vi "AutoRun.vi"() -> ()   [LabVIEW 2012]
uses:
  <vilib>/Utility/error.llb/whitespace.ctl
  resultShow.vi
panel:
  in  "布尔":bool
  in  "stepECUbracket":string
  out "毫秒计时值":u32
  in  "stepMotor/ECU":string
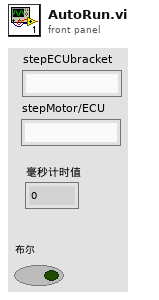
[diagram p1: front panel]
types:
  T1 = cluster{"takesTime":refnum<vi>, "userStatus":refnum<vi>, "userName":refnum<vi>, "connectionMode":refnum<vi>, "productsName":refnum<vi>, "rigStatus":refnum<vi>, "管柱码":refnum<vi>, "电机码":refnum<vi>, "控制器码":refnum<vi>, "rigStatus 2":refnum<vi>}
  T2 = typedef "whitespace.ctl" = u16
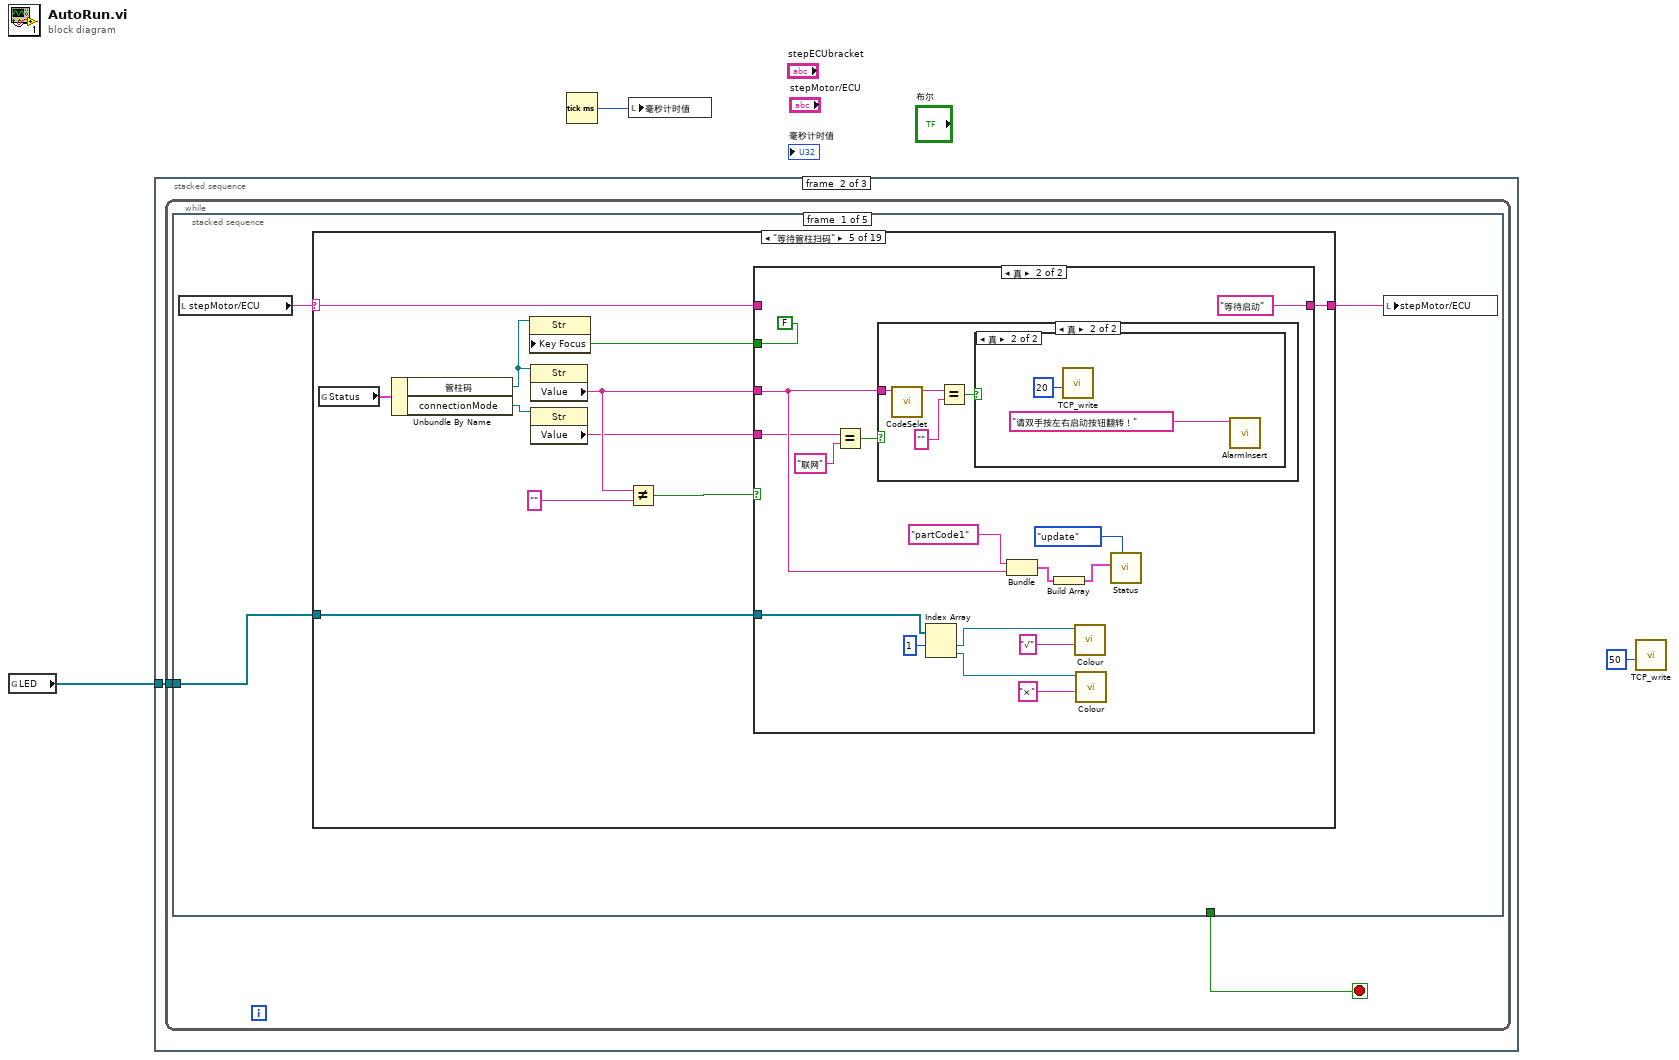
[diagram p0: block diagram]
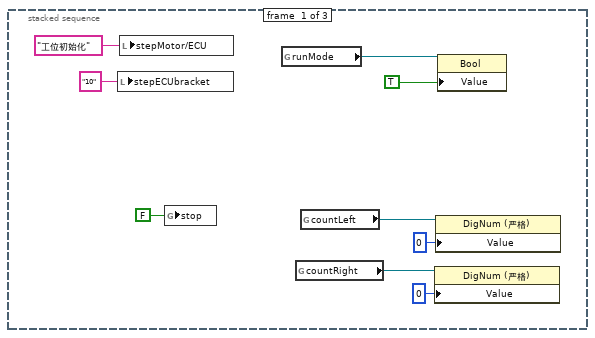
[diagram p2: hidden frame]
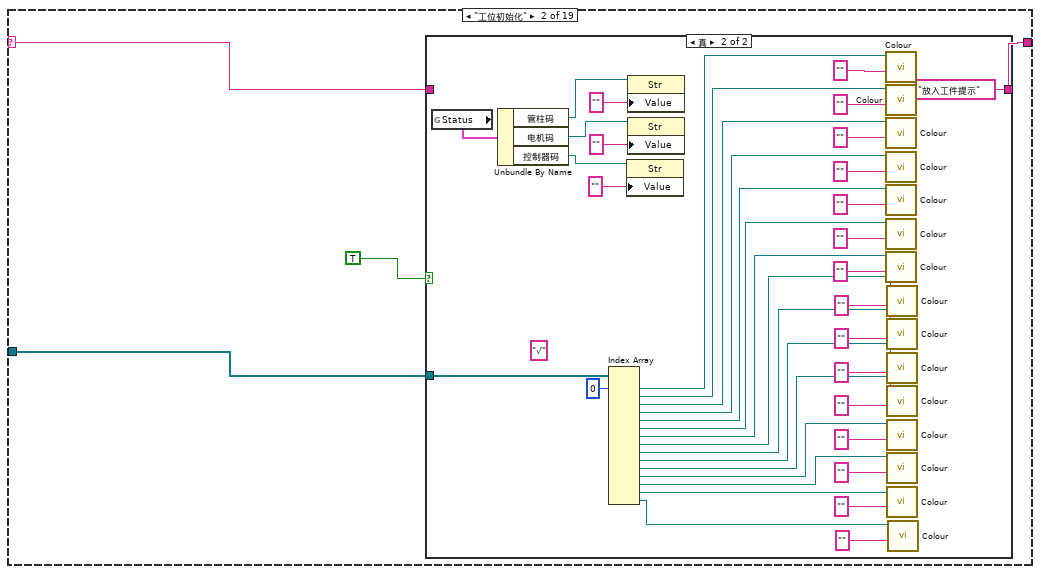
[diagram p4: hidden frame]
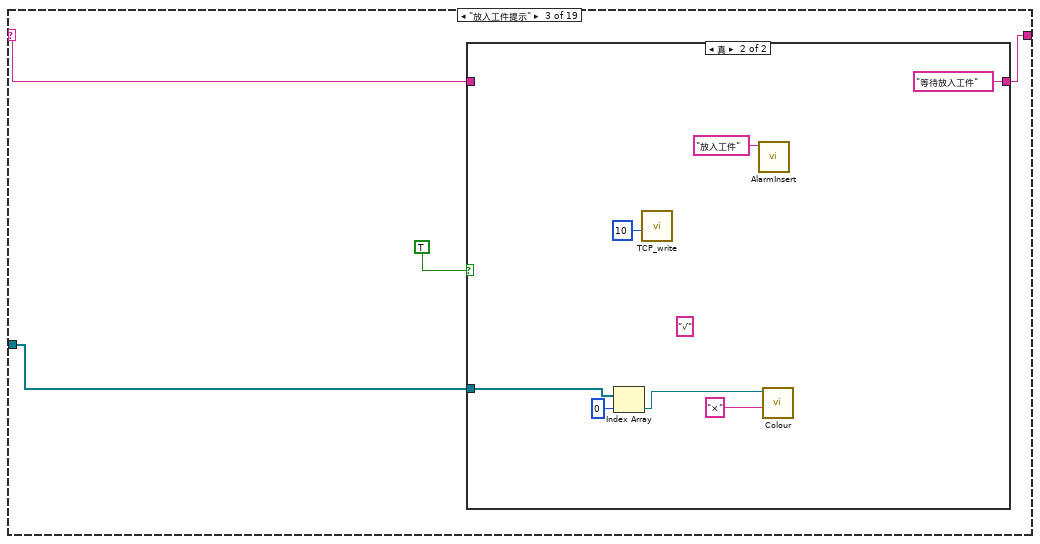
[diagram p6: hidden frame]
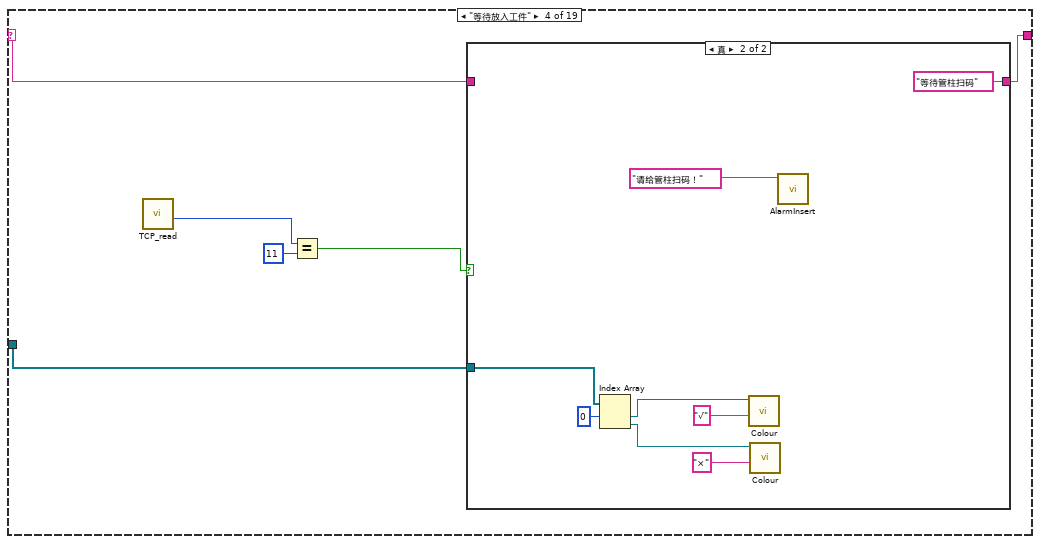
[diagram p8: hidden frame]
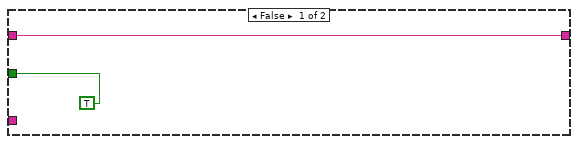
[diagram p10: hidden frame]
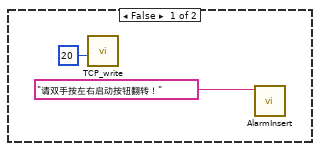
[diagram p11: hidden frame]
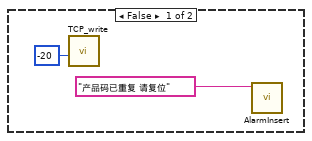
[diagram p12: hidden frame]
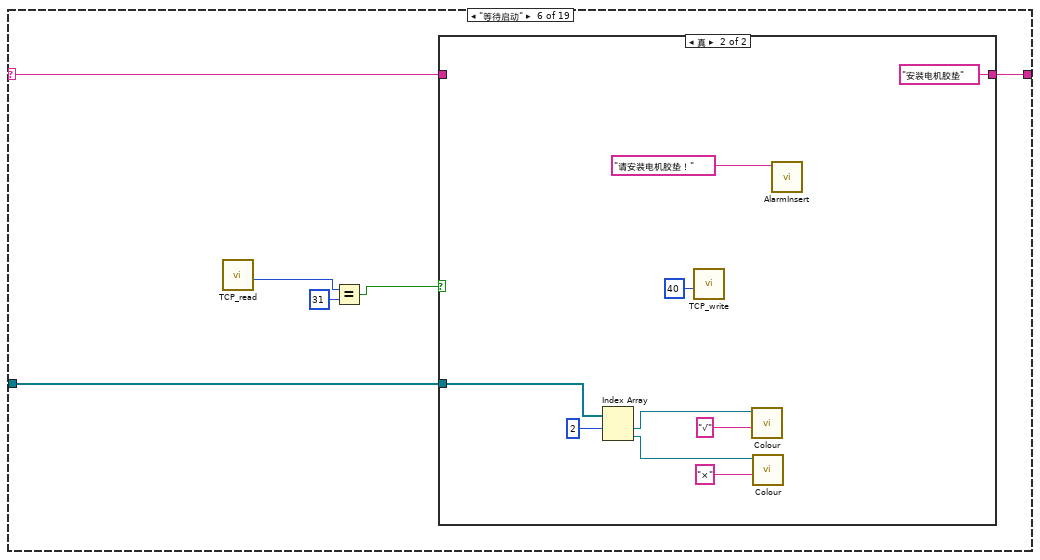
[diagram p13: hidden frame]
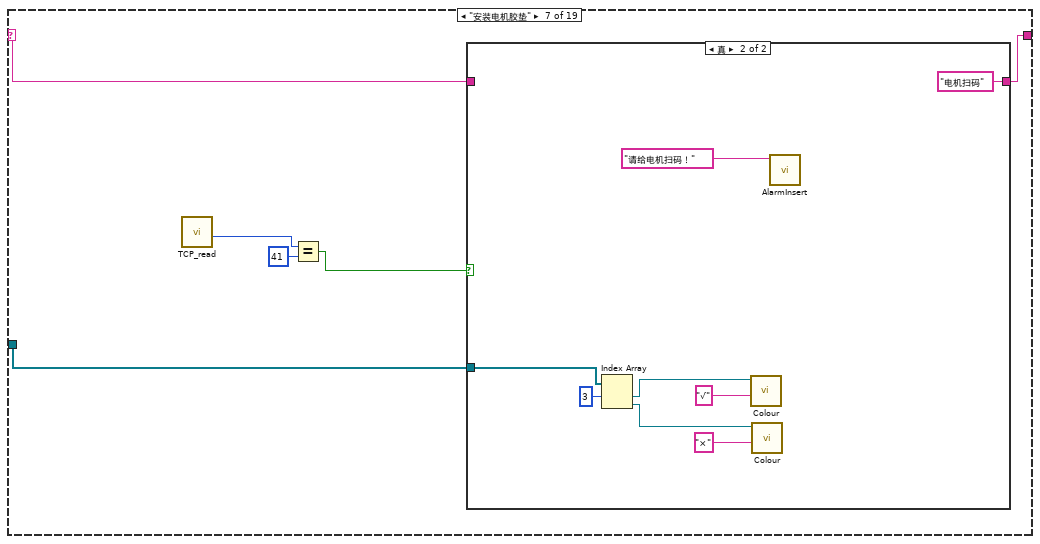
[diagram p15: hidden frame]
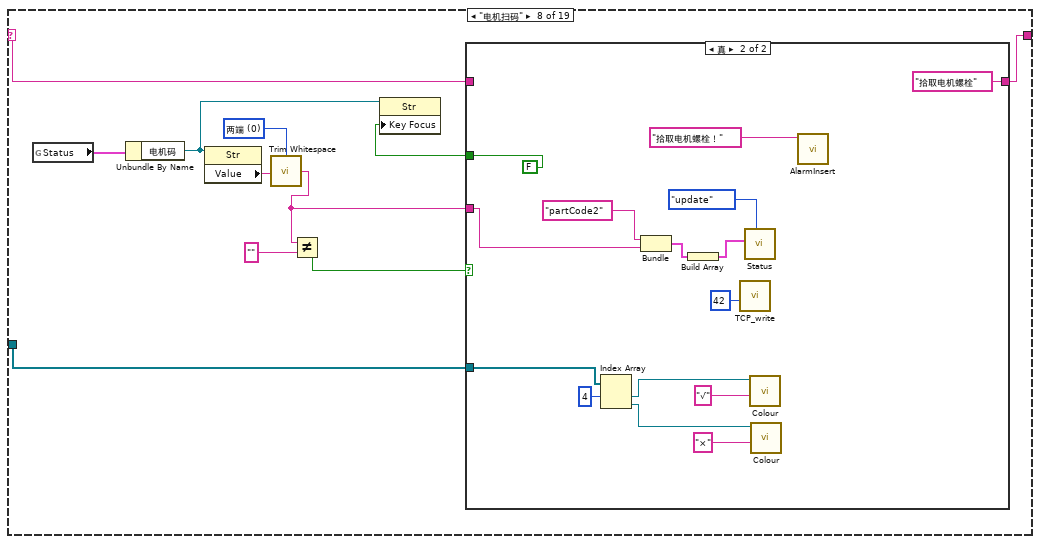
[diagram p17: hidden frame]
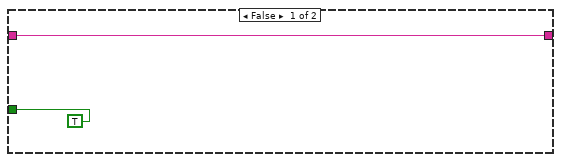
[diagram p18: hidden frame]
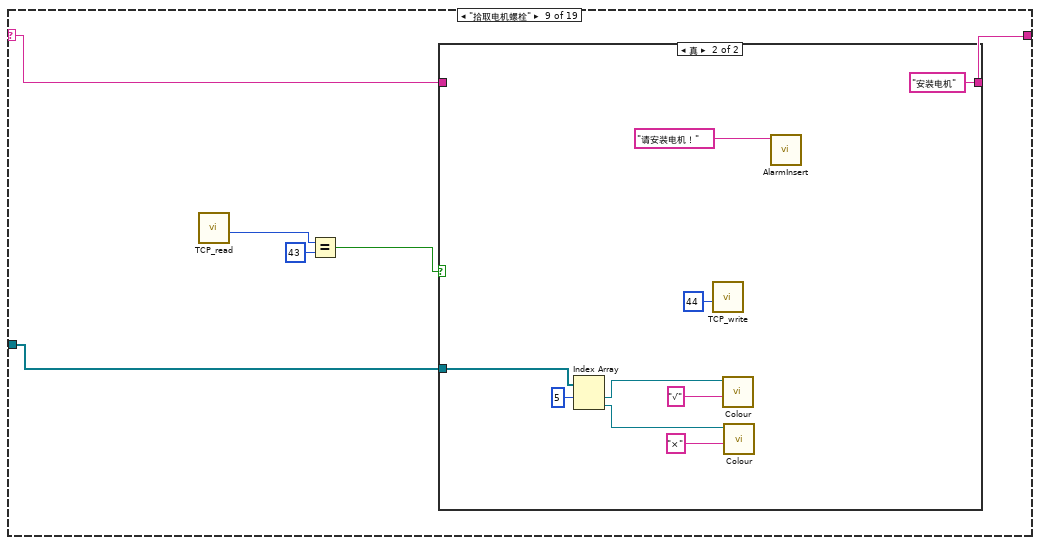
[diagram p19: hidden frame]
diagram:
  n1 = global read "resultShow.vi" "LED"() -> (w3:refnum<vi>[])
  n2 = stacked-sequence {
    tunnel: w3 -> [_ w13 _]
    frame #0 {
      n3 = local write "stepECUbracket"("10" ("step")) -> ()
      n4 = local write "stepMotor/ECU"("工位初始化" ("step")) -> ()
      n5 = global write "全局 3.vi" "stop"(FALSE ("布尔 2")) -> ()
      n6 = global read "resultShow.vi" "runMode"() -> (w9:refnum<vi>)
      n7 = global read "resultShow.vi" "countRight"() -> (w7:refnum<vi>)
      n8 = global read "resultShow.vi" "countLeft"() -> (w4:refnum<vi>)
      n9 = property class="DigNum (严格)"(reference=w7, "Value"=u32 0 ("值")) -> ()  [unwired: 1 in, 2 out]
      n10 = property class="DigNum (严格)"(reference=w4, "Value"=u32 0 ("值")) -> ()  [unwired: 1 in, 2 out]
      n11 = property class="Bool"(reference=w9, "Value"=TRUE ("m")) -> ()  [unwired: 1 in, 2 out]
    }
    frame #1 {
      n12 = while {
        tunnel: w13 -> [w14]
        stop <- w15 stop-if-true
        n13 = stacked-sequence {
          tunnel: [_ _ _ _ w510] -> w15
          tunnel: w14 -> [w17 _ _ w410 _]
          frame #0 {
            n14 = local read "stepMotor/ECU"() -> (w16:string)
            n15 = case shown="\"等待管柱扫码\"" w16 {
              selector: w16 -> [w19 w22 w67 w81 w101 w135 w151 w171 w193 w210 w224 w240 w256 w277 w299 w316 w329 w347 w370]
              tunnel: [w19 w23 w68 w82 w102 w136 w152 w169 w195 w211 w222 w238 w254 w272 w300 w315 w327 w348 w371] -> w18
              tunnel: w17 -> [_ w21 w66 w77 w100 w131 w147 w170 w194 w206 w223 w239 w255 w276 w298 w314 w328 w343 w366]
              frame "假", Default {
              }
              frame "工位初始化" {
                n16 = case shown="真" TRUE {
                  tunnel: [w24 "放入工件提示"] -> w23
                  tunnel: w22 -> [w24 _]
                  tunnel: w21 -> [_ w62]
                  frame False {
                  }
                  frame True {
                    (unwired) "√" ("元素")
                    n17 = global read "resultShow.vi" "Status"() -> (w35:T1)
                    n18 = Unbundle By Name(w35) -> ("管柱码"=w34:refnum<vi>, "电机码"=w31:refnum<vi>, "控制器码"=w29:refnum<vi>)
                    n19 = Index Array(array=w62, index #1=0 ("索引")) -> (element #1=w54:refnum<vi>, element #2=w53:refnum<vi>, element #3=w52:refnum<vi>, element #4=w51:refnum<vi>, element #5=w50:refnum<vi>, element #6=w49:refnum<vi>, element #7=w48:refnum<vi>, element #8=w41:refnum<vi>, element #9=w40:refnum<vi>, element #10=w39:refnum<vi>, element #11=w38:refnum<vi>, element #12=w37:refnum<vi>, element #13=w36:refnum<vi>, element #14=w27:refnum<vi>, element #15=w25:refnum<vi>)  [unwired: 14 in]
                    n20 = property class="Str"(reference=w29, "Value"="") -> ()  [unwired: 1 in, 2 out]
                    n21 = property class="Str"(reference=w34, "Value"="") -> ()  [unwired: 1 in, 2 out]
                    n22 = property class="Str"(reference=w31, "Value"="") -> ()  [unwired: 1 in, 2 out]
                    n23 = call "Colour.vi"("result"="" ("元素"), "colourRef"=w54) -> ()  [unwired: 9 in, 1 out]
                    n24 = call "Colour.vi"("result"="" ("元素"), "colourRef"=w53) -> ()  [unwired: 9 in, 1 out]
                    n25 = call "Colour.vi"("result"="" ("元素"), "colourRef"=w52) -> ()  [unwired: 9 in, 1 out]
                    n26 = call "Colour.vi"("result"="" ("元素"), "colourRef"=w51) -> ()  [unwired: 9 in, 1 out]
                    n27 = call "Colour.vi"("result"="" ("元素"), "colourRef"=w50) -> ()  [unwired: 9 in, 1 out]
                    n28 = call "Colour.vi"("result"="" ("元素"), "colourRef"=w49) -> ()  [unwired: 9 in, 1 out]
                    n29 = call "Colour.vi"("result"="" ("元素"), "colourRef"=w48) -> ()  [unwired: 9 in, 1 out]
                    n30 = call "Colour.vi"("result"="" ("元素"), "colourRef"=w41) -> ()  [unwired: 9 in, 1 out]
                    n31 = call "Colour.vi"("result"="" ("元素"), "colourRef"=w40) -> ()  [unwired: 9 in, 1 out]
                    n32 = call "Colour.vi"("result"="" ("元素"), "colourRef"=w39) -> ()  [unwired: 9 in, 1 out]
                    n33 = call "Colour.vi"("result"="" ("元素"), "colourRef"=w38) -> ()  [unwired: 9 in, 1 out]
                    n34 = call "Colour.vi"("result"="" ("元素"), "colourRef"=w37) -> ()  [unwired: 9 in, 1 out]
                    n35 = call "Colour.vi"("result"="" ("元素"), "colourRef"=w36) -> ()  [unwired: 9 in, 1 out]
                    n36 = call "Colour.vi"("result"="" ("元素"), "colourRef"=w27) -> ()  [unwired: 9 in, 1 out]
                    n37 = call "Colour.vi"("result"="" ("元素"), "colourRef"=w25) -> ()  [unwired: 9 in, 1 out]
                  }
                }
              }
              frame "放入工件提示" {
                n38 = case shown="真" TRUE {
                  tunnel: [w69 "等待放入工件"] -> w68
                  tunnel: w67 -> [w69 _]
                  tunnel: w66 -> [_ w72]
                  frame False {
                  }
                  frame True {
                    (unwired) "√" ("元素")
                    n39 = Index Array(array=w72, index=0 ("索引")) -> (element=w74:refnum<vi>)
                    n40 = call "TCP_write.vi"("写入数据"=i8 10) -> ()  [unwired: 11 in]
                    n41 = call "AlarmInsert.vi"("消息名"="放入工件") -> ()  [unwired: 11 in]
                    n42 = call "Colour.vi"("result"="×" ("元素"), "colourRef"=w74) -> ()  [unwired: 9 in, 1 out]
                  }
                }
              }
              frame "等待放入工件" {
                n43 = call "TCP_read.vi"() -> ("元素"=w80:i8)  [unwired: 10 in, 1 out]
                n44 = Equal?(x=w80, y=i8 11) -> (x = y?=w78:bool)
                n45 = case shown="真" w78 {
                  tunnel: [w83 "等待管柱扫码"] -> w82
                  tunnel: w81 -> [w83 _]
                  tunnel: w77 -> [_ w84]
                  frame False {
                  }
                  frame True {
                    n46 = Index Array(array=w84, index #1=0 ("索引")) -> (element #1=w88:refnum<vi>, element #2=w85:refnum<vi>)  [unwired: 1 in]
                    n47 = call "Colour.vi"("result"="√" ("元素"), "colourRef"=w88) -> ()  [unwired: 9 in, 1 out]
                    n48 = call "Colour.vi"("result"="×" ("元素"), "colourRef"=w85) -> ()  [unwired: 9 in, 1 out]
                    n49 = call "AlarmInsert.vi"("消息名"="请给管柱扫码！" ("string_5")) -> ()  [unwired: 11 in]
                  }
                }
              }
              frame "等待管柱扫码" {
                n50 = global read "resultShow.vi" "Status"() -> (w99:T1)
                n51 = Unbundle By Name(w99) -> ("管柱码"=w96:refnum<vi>, "connectionMode"=w93:refnum<vi>)
                n52 = property class="Str"(reference=w96) -> ("Value"=w94:string)  [unwired: 1 in, 2 out]
                n53 = property class="Str"(reference=w93) -> ("Value"=w92:string)  [unwired: 1 in, 2 out]
                n54 = Not Equal?(x=w94, y="") -> (x != y?=w98:bool)
                n55 = case shown="真" w98 {
                  tunnel: [w104 "等待启动"] -> w102
                  tunnel: w101 -> [w104 _]
                  tunnel: w100 -> [_ w114]
                  tunnel: [TRUE FALSE] -> w95
                  tunnel: w94 -> [_ w108]
                  tunnel: w92 -> [_ w105]
                  frame False {
                  }
                  frame True {
                    n56 = Equal?(x=w105, y="联网") -> (x = y?=w107:bool)
                    n57 = case shown="真" w107 {
                      tunnel: w108 -> [_ w126]
                      frame False {
                        n58 = call "TCP_write.vi"("写入数据"=i8 20) -> ()  [unwired: 11 in]
                        n59 = call "AlarmInsert.vi"("消息名"="请双手按左右启动按钮翻转！" ("string_5")) -> ()  [unwired: 11 in]
                      }
                      frame True {
                        n60 = call "CodeSelet.vi"("parameter name"=w126) -> ("readData"=w125:string)  [unwired: 10 in]
                        n61 = Equal?(x=w125, y="") -> (x = y?=w124:bool)
                        n62 = case shown="真" w124 {
                          frame False {
                            n63 = call "TCP_write.vi"("写入数据"=i8 -20) -> ()  [unwired: 11 in]
                            n64 = call "AlarmInsert.vi"("消息名"="产品码已重复 请复位" ("string_5")) -> ()  [unwired: 11 in]
                          }
                          frame True {
                            n65 = call "TCP_write.vi"("写入数据"=i8 20) -> ()  [unwired: 11 in]
                            n66 = call "AlarmInsert.vi"("消息名"="请双手按左右启动按钮翻转！" ("string_5")) -> ()  [unwired: 11 in]
                          }
                        }
                      }
                    }
                    n67 = Index Array(array=w114, index #1=1 ("索引")) -> (element #1=w118:refnum<vi>, element #2=w115:refnum<vi>)  [unwired: 1 in]
                    n68 = Bundle("元素"="partCode1", "Value"=w108) -> (w110:cluster{"元素":string, "Value":string})  [unwired: 1 in]
                    n69 = Build Array(w110) -> (w111:cluster{"元素":string, "Value":string}[])
                    n70 = call "Colour.vi"("result"="√" ("元素"), "colourRef"=w118) -> ()  [unwired: 9 in, 1 out]
                    n71 = call "Colour.vi"("result"="×" ("元素"), "colourRef"=w115) -> ()  [unwired: 9 in, 1 out]
                    n72 = call "Status.vi"("模式"=enum16{"select", "insert", "update", "delete"}."update", "nameData"=w111) -> ()  [unwired: 9 in, 1 out]
                  }
                }
                n73 = property class="Str"(reference=w96, "Key Focus"=w95) -> ()  [unwired: 1 in, 2 out]
              }
              frame "等待启动" {
                n74 = call "TCP_read.vi"() -> ("元素"=w134:i8)  [unwired: 10 in, 1 out]
                n75 = Equal?(x=w134, y=i8 31) -> (x = y?=w132:bool)
                n76 = case shown="真" w132 {
                  tunnel: [w137 "安装电机胶垫"] -> w136
                  tunnel: w135 -> [w137 _]
                  tunnel: w131 -> [_ w139]
                  frame False {
                  }
                  frame True {
                    n77 = Index Array(array=w139, index #1=2 ("索引")) -> (element #1=w143:refnum<vi>, element #2=w140:refnum<vi>)  [unwired: 1 in]
                    n78 = call "TCP_write.vi"("写入数据"=i8 40) -> ()  [unwired: 11 in]
                    n79 = call "Colour.vi"("result"="√" ("元素"), "colourRef"=w143) -> ()  [unwired: 9 in, 1 out]
                    n80 = call "Colour.vi"("result"="×" ("元素"), "colourRef"=w140) -> ()  [unwired: 9 in, 1 out]
                    n81 = call "AlarmInsert.vi"("消息名"="请安装电机胶垫！" ("string_5")) -> ()  [unwired: 11 in]
                  }
                }
              }
              frame "安装电机胶垫" {
                n82 = call "TCP_read.vi"() -> ("元素"=w150:i8)  [unwired: 10 in, 1 out]
                n83 = Equal?(x=w150, y=i8 41) -> (x = y?=w148:bool)
                n84 = case shown="真" w148 {
                  tunnel: [w153 "电机扫码"] -> w152
                  tunnel: w151 -> [w153 _]
                  tunnel: w147 -> [_ w154]
                  frame False {
                  }
                  frame True {
                    n85 = Index Array(array=w154, index #1=3 ("索引")) -> (element #1=w158:refnum<vi>, element #2=w155:refnum<vi>)  [unwired: 1 in]
                    n86 = call "Colour.vi"("result"="√" ("元素"), "colourRef"=w158) -> ()  [unwired: 9 in, 1 out]
                    n87 = call "Colour.vi"("result"="×" ("元素"), "colourRef"=w155) -> ()  [unwired: 9 in, 1 out]
                    n88 = call "AlarmInsert.vi"("消息名"="请给电机扫码！" ("string_5")) -> ()  [unwired: 11 in]
                  }
                }
              }
              frame "电机扫码" {
                w162 = T2 0 items=["两端", "字符串首端", "字符串末端"] ("location (both)")
                n89 = global read "resultShow.vi" "Status"() -> (w167:T1)
                n90 = Unbundle By Name(w167) -> ("电机码"=w166:refnum<vi>)
                n91 = property class="Str"(reference=w166) -> ("Value"=w164:string)  [unwired: 1 in, 2 out]
                n92 = call <vilib>:"Trim Whitespace.vi"("string"=w164, "location (both)"=w162) -> ("trimmed string"=w163:string)
                n93 = Not Equal?(x=w163, y="") -> (x != y?=w172:bool)
                n94 = case shown="真" w172 {
                  tunnel: [w174 "拾取电机螺栓"] -> w169
                  tunnel: w171 -> [w174 _]
                  tunnel: w170 -> [_ w181]
                  tunnel: [TRUE FALSE] -> w165
                  tunnel: w163 -> [_ w175]
                  frame False {
                  }
                  frame True {
                    n95 = Index Array(array=w181, index #1=4 ("索引")) -> (element #1=w185:refnum<vi>, element #2=w182:refnum<vi>)  [unwired: 1 in]
                    n96 = Bundle("元素"="partCode2", "trimmed string"=w175) -> (w177:cluster{"元素":string, "trimmed string":string})  [unwired: 1 in]
                    n97 = Build Array(w177) -> (w178:cluster{"元素":string, "trimmed string":string}[])
                    n98 = call "TCP_write.vi"("写入数据"=i8 42) -> ()  [unwired: 11 in]
                    n99 = call "Status.vi"("模式"=enum16{"select", "insert", "update", "delete"}."update", "nameData"=w178) -> ()  [unwired: 9 in, 1 out]
                    n100 = call "Colour.vi"("result"="√" ("元素"), "colourRef"=w185) -> ()  [unwired: 9 in, 1 out]
                    n101 = call "Colour.vi"("result"="×" ("元素"), "colourRef"=w182) -> ()  [unwired: 9 in, 1 out]
                    n102 = call "AlarmInsert.vi"("消息名"="拾取电机螺栓！" ("string_5")) -> ()  [unwired: 11 in]
                  }
                }
                n103 = property class="Str"(reference=w166, "Key Focus"=w165) -> ()  [unwired: 1 in, 2 out]
              }
              frame "拾取电机螺栓" {
                n104 = call "TCP_read.vi"() -> ("元素"=w192:i8)  [unwired: 10 in, 1 out]
                n105 = Equal?(x=w192, y=i8 43) -> (x = y?=w190:bool)
                n106 = case shown="真" w190 {
                  tunnel: [w196 "安装电机"] -> w195
                  tunnel: w193 -> [w196 _]
                  tunnel: w194 -> [_ w197]
                  frame False {
                  }
                  frame True {
                    n107 = Index Array(array=w197, index #1=5 ("索引")) -> (element #1=w201:refnum<vi>, element #2=w198:refnum<vi>)  [unwired: 1 in]
                    n108 = call "TCP_write.vi"("写入数据"=i8 44) -> ()  [unwired: 11 in]
                    n109 = call "Colour.vi"("result"="√" ("元素"), "colourRef"=w201) -> ()  [unwired: 9 in, 1 out]
                    n110 = call "Colour.vi"("result"="×" ("元素"), "colourRef"=w198) -> ()  [unwired: 9 in, 1 out]
                    n111 = call "AlarmInsert.vi"("消息名"="请安装电机！" ("string_5")) -> ()  [unwired: 11 in]
                  }
                }
              }
              frame "安装电机" {
                n112 = call "TCP_read.vi"() -> ("元素"=w209:i8)  [unwired: 10 in, 1 out]
                n113 = Equal?(x=w209, y=i8 45) -> (x = y?=w207:bool)
                n114 = case shown="真" w207 {
                  tunnel: [w212 "涂电机色标"] -> w211
                  tunnel: w210 -> [w212 _]
                  tunnel: w206 -> [_ w213]
                  frame False {
                  }
                  frame True {
                    n115 = Index Array(array=w213, index #1=6 ("索引")) -> (element #1=w217:refnum<vi>, element #2=w214:refnum<vi>)  [unwired: 1 in]
                    n116 = call "TCP_write.vi"("写入数据"=i8 46) -> ()  [unwired: 11 in]
                    n117 = call "Colour.vi"("result"="√" ("元素"), "colourRef"=w217) -> ()  [unwired: 9 in, 1 out]
                    n118 = call "Colour.vi"("result"="×" ("元素"), "colourRef"=w214) -> ()  [unwired: 9 in, 1 out]
                    n119 = call "AlarmInsert.vi"("消息名"="请涂电机色标！" ("string_5")) -> ()  [unwired: 11 in]
                  }
                }
              }
              frame "涂电机色标" {
                n120 = call "TCP_read.vi"() -> ("元素"=w227:i8)  [unwired: 10 in, 1 out]
                n121 = Equal?(x=w227, y=i8 47) -> (x = y?=w225:bool)
                n122 = case shown="真" w225 {
                  tunnel: [w228 "启动平翻"] -> w222
                  tunnel: w224 -> [w228 _]
                  tunnel: w223 -> [_ w229]
                  frame False {
                  }
                  frame True {
                    n123 = Index Array(array=w229, index #1=7 ("索引")) -> (element #1=w233:refnum<vi>, element #2=w230:refnum<vi>)  [unwired: 1 in]
                    n124 = call "TCP_write.vi"("写入数据"=i8 50) -> ()  [unwired: 11 in]
                    n125 = call "Colour.vi"("result"="√" ("元素"), "colourRef"=w233) -> ()  [unwired: 9 in, 1 out]
                    n126 = call "Colour.vi"("result"="×" ("元素"), "colourRef"=w230) -> ()  [unwired: 9 in, 1 out]
                    n127 = call "AlarmInsert.vi"("消息名"="请双手按启动按钮翻转至平位" ("string_5")) -> ()  [unwired: 11 in]
                  }
                }
              }
              frame "启动平翻" {
                n128 = call "TCP_read.vi"() -> ("元素"=w241:i8)  [unwired: 10 in, 1 out]
                n129 = Equal?(x=w241, y=i8 53) -> (x = y?=w243:bool)
                n130 = case shown="真" w243 {
                  tunnel: [w244 "防错确认"] -> w238
                  tunnel: w240 -> [w244 _]
                  tunnel: w239 -> [_ w246]
                  frame False {
                  }
                  frame True {
                    n131 = Index Array(array=w246, index #1=8 ("索引")) -> (element #1=w250:refnum<vi>, element #2=w247:refnum<vi>)  [unwired: 1 in]
                    n132 = call "Colour.vi"("result"="√" ("元素"), "colourRef"=w250) -> ()  [unwired: 9 in, 1 out]
                    n133 = call "Colour.vi"("result"="×" ("元素"), "colourRef"=w247) -> ()  [unwired: 9 in, 1 out]
                    n134 = call "TCP_write.vi"("写入数据"=i8 90) -> ()  [unwired: 11 in]
                    n135 = call "AlarmInsert.vi"("消息名"="防错确认" ("string_5")) -> ()  [unwired: 11 in]
                  }
                }
              }
              frame "防错确认" {
                n136 = call "TCP_read.vi"() -> ("元素"=w257:i8)  [unwired: 10 in, 1 out]
                n137 = Equal?(x=w257, y=i8 91) -> (x = y?=w259:bool)
                n138 = case shown="真" w259 {
                  tunnel: [w260 "控制器扫码"] -> w254
                  tunnel: w256 -> [w260 _]
                  tunnel: w255 -> [_ w261]
                  frame False {
                  }
                  frame True {
                    n139 = Index Array(array=w261, index #1=9 ("索引")) -> (element #1=w265:refnum<vi>, element #2=w262:refnum<vi>)  [unwired: 1 in]
                    n140 = call "Colour.vi"("result"="√" ("元素"), "colourRef"=w265) -> ()  [unwired: 9 in, 1 out]
                    n141 = call "Colour.vi"("result"="×" ("元素"), "colourRef"=w262) -> ()  [unwired: 9 in, 1 out]
                    n142 = call "AlarmInsert.vi"("消息名"="取控制器扫码" ("string_5")) -> ()  [unwired: 11 in]
                  }
                }
              }
              frame "控制器扫码" {
                n143 = global read "resultShow.vi" "Status"() -> (w274:T1)
                n144 = Unbundle By Name(w274) -> ("控制器码"=w271:refnum<vi>)
                n145 = property class="Str"(reference=w271) -> ("Value"=w269:string)  [unwired: 1 in, 2 out]
                n146 = Not Equal?(x=w269, y="") -> (x != y?=w273:bool)
                n147 = case shown="真" w273 {
                  tunnel: [w279 "拾取控制器螺栓"] -> w272
                  tunnel: w277 -> [w279 _]
                  tunnel: w276 -> [_ w287]
                  tunnel: [TRUE FALSE] -> w270
                  tunnel: w269 -> [_ w280]
                  frame False {
                  }
                  frame True {
                    n148 = Index Array(array=w287, index #1=10 ("索引")) -> (element #1=w291:refnum<vi>, element #2=w288:refnum<vi>)  [unwired: 1 in]
                    n149 = Bundle("元素"="partCode3", "Value"=w280) -> (w282:cluster{"元素":string, "Value":string})  [unwired: 1 in]
                    n150 = Build Array(w282) -> (w283:cluster{"元素":string, "Value":string}[])
                    n151 = call "Colour.vi"("result"="√" ("元素"), "colourRef"=w291) -> ()  [unwired: 9 in, 1 out]
                    n152 = call "Colour.vi"("result"="×" ("元素"), "colourRef"=w288) -> ()  [unwired: 9 in, 1 out]
                    n153 = call "TCP_write.vi"("写入数据"=i8 54) -> ()  [unwired: 11 in]
                    n154 = call "Status.vi"("模式"=enum16{"select", "insert", "update", "delete"}."update", "nameData"=w283) -> ()  [unwired: 9 in, 1 out]
                    n155 = call "AlarmInsert.vi"("消息名"="拾取控制器螺栓" ("string_5")) -> ()  [unwired: 11 in]
                  }
                }
                n156 = property class="Str"(reference=w271, "Key Focus"=w270) -> ()  [unwired: 1 in, 2 out]
              }
              frame "拾取控制器螺栓" {
                n157 = call "TCP_read.vi"() -> ("元素"=w296:i8)  [unwired: 10 in, 1 out]
                n158 = Equal?(x=w296, y=i8 55) -> (x = y?=w295:bool)
                n159 = case shown="真" w295 {
                  tunnel: [w301 "安装控制器"] -> w300
                  tunnel: w299 -> [w301 _]
                  tunnel: w298 -> [_ w303]
                  frame False {
                  }
                  frame True {
                    n160 = Index Array(array=w303, index #1=11 ("索引")) -> (element #1=w307:refnum<vi>, element #2=w304:refnum<vi>)  [unwired: 1 in]
                    n161 = call "TCP_write.vi"("写入数据"=i8 56) -> ()  [unwired: 11 in]
                    n162 = call "Colour.vi"("result"="√" ("元素"), "colourRef"=w307) -> ()  [unwired: 9 in, 1 out]
                    n163 = call "Colour.vi"("result"="×" ("元素"), "colourRef"=w304) -> ()  [unwired: 9 in, 1 out]
                    n164 = call "AlarmInsert.vi"("消息名"="请安装控制器" ("string_5")) -> ()  [unwired: 11 in]
                  }
                }
              }
              frame "安装控制器" {
                n165 = call "TCP_read.vi"() -> ("元素"=w312:i8)  [unwired: 10 in, 1 out]
                n166 = Equal?(x=w312, y=i8 57) -> (x = y?=w311:bool)
                n167 = case shown="真" w311 {
                  tunnel: [w317 "涂控制器色标"] -> w315
                  tunnel: w316 -> [w317 _]
                  tunnel: w314 -> [_ w319]
                  frame False {
                  }
                  frame True {
                    n168 = Index Array(array=w319, index #1=12 ("索引")) -> (element #1=w323:refnum<vi>, element #2=w320:refnum<vi>)  [unwired: 1 in]
                    n169 = call "TCP_write.vi"("写入数据"=i8 60) -> ()  [unwired: 11 in]
                    n170 = call "Colour.vi"("result"="√" ("元素"), "colourRef"=w323) -> ()  [unwired: 9 in, 1 out]
                    n171 = call "Colour.vi"("result"="×" ("元素"), "colourRef"=w320) -> ()  [unwired: 9 in, 1 out]
                    n172 = call "AlarmInsert.vi"("消息名"="请涂控制器螺钉色标" ("string_5")) -> ()  [unwired: 11 in]
                  }
                }
              }
              frame "涂控制器色标" {
                n173 = call "TCP_read.vi"() -> ("元素"=w331:i8)  [unwired: 10 in, 1 out]
                n174 = Equal?(x=w331, y=i8 61) -> (x = y?=w330:bool)
                n175 = case shown="真" w330 {
                  tunnel: [w333 "80"] -> w327
                  tunnel: w329 -> [w333 _]
                  tunnel: w328 -> [_ w335]
                  frame False {
                  }
                  frame True {
                    n176 = Index Array(array=w335, index #1=13 ("索引")) -> (element #1=w339:refnum<vi>, element #2=w336:refnum<vi>)  [unwired: 1 in]
                    n177 = call "TCP_write.vi"("写入数据"=i8 70) -> ()  [unwired: 11 in]
                    n178 = call "Colour.vi"("result"="√" ("元素"), "colourRef"=w339) -> ()  [unwired: 9 in, 1 out]
                    n179 = call "Colour.vi"("result"="×" ("元素"), "colourRef"=w336) -> ()  [unwired: 9 in, 1 out]
                    n180 = call "AlarmInsert.vi"("消息名"="请取出工件" ("string_5")) -> ()  [unwired: 11 in]
                  }
                }
              }
              frame "80" {
                n181 = call "TCP_read.vi"() -> ("元素"=w346:i8)  [unwired: 10 in, 1 out]
                n182 = Equal?(x=w346, y=i8 71) -> (x = y?=w344:bool)
                n183 = case shown="真" w344 {
                  tunnel: [w349 "90"] -> w348
                  tunnel: w347 -> [w349 _]
                  tunnel: w343 -> [_ w350]
                  frame False {
                  }
                  frame True {
                    n184 = local read "毫秒计时值"() -> (w357:u32)
                    n185 = Tick Count (ms)() -> (millisecond timer value=w362:u32)
                    n186 = Index Array(array=w350, index #1=13 ("索引")) -> (element #1=w354:refnum<vi>, element #2=w351:refnum<vi>)  [unwired: 1 in]
                    n187 = Subtract(x=w362, y=w357) -> (x-y=w361:u32)
                    n188 = Divide(x=w361, y=u32 1000) -> (x/y=w359:dbl)
                    n189 = To Time Stamp(1:w359) -> (0:w358:timestamp)
                    n190 = call "Colour.vi"("result"="√" ("元素"), "colourRef"=w354) -> ()  [unwired: 9 in, 1 out]
                    n191 = call "Colour.vi"("result"="×" ("元素"), "colourRef"=w351) -> ()  [unwired: 9 in, 1 out]
                    n192 = Format Date/Time String(seconds (now)=w358) -> (date/time string=w356:string)  [unwired: 2 in]
                    n193 = call "TCP_write.vi"("写入数据"=i8 80) -> ()  [unwired: 11 in]
                    n194 = call "AlarmInsert.vi"("takesTime"=w356, "消息名"="完成取回工件！" ("string_5")) -> ()  [unwired: 10 in]
                  }
                }
              }
              frame "90" {
                n195 = call "TCP_read.vi"() -> ("元素"=w369:i8)  [unwired: 10 in, 1 out]
                n196 = Equal?(x=w369, y=i8 81) -> (x = y?=w367:bool)
                n197 = case shown="真" w367 {
                  tunnel: [w372 "工位初始化"] -> w371
                  tunnel: w370 -> [w372 _]
                  tunnel: w366 -> [_ w382]
                  frame False {
                  }
                  frame True {
                    n198 = global read "resultShow.vi" "Status"() -> (w376:T1)
                    n199 = global read "resultShow.vi" "countLeft"() -> (w381:refnum<vi>)
                    n200 = Unbundle By Name(w376) -> ("connectionMode"=w377:refnum<vi>)
                    n201 = Index Array(array=w382, index=14 ("索引")) -> (element=w384:refnum<vi>)
                    n202 = property class="DigNum (严格)"(reference=w381) -> (reference out=w380:refnum<vi>, "Value"=w379:u32)  [unwired: 1 in, 1 out]
                    n203 = property class="Str"(reference=w377) -> ("Value"=w374:string)  [unwired: 1 in, 2 out]
                    n204 = call "Colour.vi"("result"="√" ("元素"), "colourRef"=w384) -> ()  [unwired: 9 in, 1 out]
                    n205 = Equal?(x=w374, y="联网") -> (x = y?=w375:bool)
                    n206 = Increment(x=w379) -> (x+1=w378:u32)
                    n207 = case shown="真" w375 {
                      frame False {
                      }
                      frame True {
                        n208 = call "Upload.vi"() -> ()  [unwired: 12 in]
                      }
                    }
                    n209 = property class="DigNum (严格)"(reference=w380, "Value"=w378) -> ()  [unwired: 1 in, 2 out]
                  }
                }
              }
            }
            n210 = local write "stepMotor/ECU"(w18) -> ()
          }
          frame #1 {
            n211 = local read "stepECUbracket"() -> (w388:string)
            n212 = global read "resultShow.vi" "runMode 2"() -> (w389:bool)
            n213 = case shown="真" w389 {
              tunnel: ["10" w391] -> w387
              tunnel: w388 -> [_ w391]
              frame False {
              }
              frame True {
              }
            }
            n214 = local write "stepECUbracket"(w387) -> ()
          }
          frame #2 {
            n215 = call "TCP_read.vi"() -> ("元素"=w396:i8)  [unwired: 10 in, 1 out]
            n216 = local read "布尔"() -> (w392:bool)
            n217 = local read "stepMotor/ECU"() -> (w398:string)
            n218 = Equal?(x=w396, y=i8 -100) -> (x = y?=w394:bool)
            n219 = Or(x=w394, y=w392) -> (x .or. y?=w393:bool)
            n220 = case shown="真" w393 {
              tunnel: [w399 w406] -> w397
              tunnel: w398 -> [w399 w401]
              frame False {
              }
              frame True {
                n221 = call "TCP_read.vi"() -> ("元素"=w404:i8)  [unwired: 10 in, 1 out]
                n222 = local write "布尔"(TRUE) -> ()
                n223 = Equal?(x=w404, y=i8 0) -> (x = y?=w402:bool)
                n224 = call "AlarmInsert.vi"("消息名"="复位中") -> ()  [unwired: 11 in]
                n225 = case shown="真" w402 {
                  tunnel: [w407 "工位初始化"] -> w406
                  tunnel: w401 -> [w407 _]
                  frame False {
                  }
                  frame True {
                    n226 = local write "布尔"(FALSE) -> ()
                  }
                }
              }
            }
            n227 = local write "stepMotor/ECU"(w397) -> ()
          }
          frame #3 {
            n228 = local read "stepECUbracket"() -> (w411:string)
            n229 = case shown="\"假\", 默认" w411 {
              selector: w411 -> [w413 w416 w438 w458 w478 w487 w492 w497 w501]
              tunnel: [w413 w417 w439 w459 w479 w488 w493 w498 w502] -> w412
              tunnel: w410 -> [_ w414 w433 w453 w473 _ _ _ _]
              frame "假", Default {
              }
              frame "10" {
                n230 = case shown="真" TRUE {
                  tunnel: [w418 "20"] -> w417
                  tunnel: w416 -> [w418 _]
                  tunnel: w414 -> [_ w424]
                  frame False {
                  }
                  frame True {
                    (unwired) "×" ("元素")
                    (unwired) "√" ("元素")
                    n231 = global read "resultShow.vi" "Status"() -> (w421:T1)
                    n232 = Unbundle By Name(w421) -> ("rigStatus 2"=w420:refnum<vi>)
                    n233 = Index Array(array=w424, index #1=15 ("索引")) -> (element #1=w428:refnum<vi>, element #2=w425:refnum<vi>, element #3=w422:refnum<vi>)  [unwired: 2 in]
                    n234 = property class="Str"(reference=w420, "Value"="请摄取控制器支架螺栓" ("string_5")) -> ()  [unwired: 1 in, 2 out]
                    n235 = call "TCP_write.vi"("写入地址"=u32 20, "写入数据"=i8 10) -> ()  [unwired: 10 in]
                    n236 = call "Colour.vi"("result"="×" ("元素"), "colourRef"=w428) -> ()  [unwired: 9 in, 1 out]
                    n237 = call "Colour.vi"("result"="" ("元素"), "colourRef"=w425) -> ()  [unwired: 9 in, 1 out]
                    n238 = call "Colour.vi"("result"="" ("元素"), "colourRef"=w422) -> ()  [unwired: 9 in, 1 out]
                  }
                }
              }
              frame "20" {
                n239 = call "TCP_read.vi"("起始地址"=u32 20) -> ("元素"=w437:i8)  [unwired: 9 in, 1 out]
                n240 = Equal?(x=w437, y=i8 11) -> (x = y?=w435:bool)
                n241 = case shown="真" w435 {
                  tunnel: [w440 "30"] -> w439
                  tunnel: w438 -> [w440 _]
                  tunnel: w433 -> [_ w447]
                  frame False {
                  }
                  frame True {
                    n242 = global read "resultShow.vi" "Status"() -> (w443:T1)
                    n243 = Index Array(array=w447, index #1=15 ("索引")) -> (element #1=w446:refnum<vi>, element #2=w444:refnum<vi>)  [unwired: 1 in]
                    n244 = Unbundle By Name(w443) -> ("rigStatus 2"=w442:refnum<vi>)
                    n245 = call "TCP_write.vi"("写入地址"=u32 20, "写入数据"=i8 20) -> ()  [unwired: 10 in]
                    n246 = call "Colour.vi"("result"="√" ("元素"), "colourRef"=w446) -> ()  [unwired: 9 in, 1 out]
                    n247 = call "Colour.vi"("result"="×" ("元素"), "colourRef"=w444) -> ()  [unwired: 9 in, 1 out]
                    n248 = property class="Str"(reference=w442, "Value"="请气枪安装控制器支架" ("string_5")) -> ()  [unwired: 1 in, 2 out]
                  }
                }
              }
              frame "30" {
                n249 = call "TCP_read.vi"("起始地址"=u32 20) -> ("元素"=w457:i8)  [unwired: 9 in, 1 out]
                n250 = Equal?(x=w457, y=i8 21) -> (x = y?=w455:bool)
                n251 = case shown="真" w455 {
                  tunnel: [w460 "40"] -> w459
                  tunnel: w458 -> [w460 _]
                  tunnel: w453 -> [_ w467]
                  frame False {
                  }
                  frame True {
                    n252 = global read "resultShow.vi" "Status"() -> (w463:T1)
                    n253 = Unbundle By Name(w463) -> ("rigStatus 2"=w462:refnum<vi>)
                    n254 = Index Array(array=w467, index #1=16 ("索引")) -> (element #1=w469:refnum<vi>, element #2=w464:refnum<vi>)  [unwired: 1 in]
                    n255 = property class="Str"(reference=w462, "Value"="请涂色标" ("string_5")) -> ()  [unwired: 1 in, 2 out]
                    n256 = call "TCP_write.vi"("写入地址"=u32 20, "写入数据"=i8 30) -> ()  [unwired: 10 in]
                    n257 = call "Colour.vi"("result"="√" ("元素"), "colourRef"=w469) -> ()  [unwired: 9 in, 1 out]
                    n258 = call "Colour.vi"("result"="×" ("元素"), "colourRef"=w464) -> ()  [unwired: 9 in, 1 out]
                  }
                }
              }
              frame "40" {
                n259 = call "TCP_read.vi"("起始地址"=u32 20) -> ("元素"=w477:i8)  [unwired: 9 in, 1 out]
                n260 = Equal?(x=w477, y=i8 31) -> (x = y?=w474:bool)
                n261 = case shown="真" w474 {
                  tunnel: [w480 "50"] -> w479
                  tunnel: w478 -> [w480 _]
                  tunnel: w473 -> [_ w481]
                  frame False {
                  }
                  frame True {
                    n262 = Index Array(array=w481, index=17 ("索引")) -> (element=w483:refnum<vi>)
                    n263 = call "Colour.vi"("result"="√" ("元素"), "colourRef"=w483) -> ()  [unwired: 9 in, 1 out]
                  }
                }
              }
              frame "50" {
                n264 = case shown="真" TRUE {
                  tunnel: [w489 "60"] -> w488
                  tunnel: w487 -> [w489 _]
                  frame False {
                  }
                  frame True {
                  }
                }
              }
              frame "60" {
                n265 = case shown="真" TRUE {
                  tunnel: [w494 "70"] -> w493
                  tunnel: w492 -> [w494 _]
                  frame False {
                  }
                  frame True {
                  }
                }
              }
              frame "70" {
                n266 = case shown="真" TRUE {
                  tunnel: [w499 "80"] -> w498
                  tunnel: w497 -> [w499 _]
                  frame False {
                  }
                  frame True {
                  }
                }
              }
              frame "80" {
                n267 = case shown="真" TRUE {
                  tunnel: [w504 "10"] -> w502
                  tunnel: w501 -> [w504 _]
                  frame False {
                  }
                  frame True {
                    n268 = global read "resultShow.vi" "countRight"() -> (w508:refnum<vi>)
                    n269 = property class="DigNum (严格)"(reference=w508) -> (reference out=w507:refnum<vi>, "Value"=w506:u32)  [unwired: 1 in, 1 out]
                    n270 = Increment(x=w506) -> (x+1=w505:u32)
                    n271 = property class="DigNum (严格)"(reference=w507, "Value"=w505) -> ()  [unwired: 1 in, 2 out]
                  }
                }
              }
            }
            n272 = local write "stepECUbracket"(w412) -> ()
          }
          frame #4 {
            n273 = global read "全局 3.vi" "stop"() -> (w510:bool)
            n274 = Wait (ms)(milliseconds to wait=u32 10 ("等待时间（毫秒）")) -> ()  [unwired: 1 out]
          }
        }
      }
    }
    frame #2 {
      n275 = global read "resultShow.vi" "runMode"() -> (w513:refnum<vi>)
      n276 = property class="Bool"(reference=w513, "Value"=FALSE ("m")) -> ()  [unwired: 1 in, 2 out]
    }
  }
  n277 = Tick Count (ms)() -> (millisecond timer value=w2:u32)
  n278 = local write "毫秒计时值"(w2) -> ()
  n279 = call "TCP_write.vi"("写入数据"=i8 50) -> ()  [unwired: 11 in]
